vi "Actor Core.vi"(8 "error in":errorcluster, 11 "Jobber in":refnum<class "Jobber.lvclass">) -> (0 "error out":errorcluster, 3 "Actor out":refnum<class "Actor.lvclass">)   [LabVIEW 2014, in "Jobber.lvlib" / "Jobber.lvclass"]
doc: "(<B>Filename</B>: Actor Framework.lvlib:Actor.lvclass:Actor Core.vi)\n\nReceives messages to the actor, reacts to them, and initiates any error handling that may shut the actor down.\n\nDescendant classes may override this VI to append parallel tasks for the actor to complete while it handles messages. Overrides use the Call Parent Method node."
uses:
  Jobber.lvclass
  <vilib>/ActorFramework/Actor/Actor.lvclass
  <vilib>/ActorFramework/Actor/Actor.lvclass/Actor.ctl
  <vilib>/ActorFramework/Message Enqueuer/Message Enqueuer.lvclass/Message Enqueuer.ctl
  Jobber.lvclass/Jobber.ctl
  Shared/Classes/Status Updater/Status Updater.lvclass/Status Updater.ctl
  Jobber Messages/Job Done Msg/Job Done Msg.lvclass/Job Done Msg.ctl
  <vilib>/ActorFramework/Message Enqueuer/Init from Existing Queue.vi
  <vilib>/ActorFramework/Message Enqueuer/Enqueue.vi
  <vilib>/ActorFramework/Message Priority Queue/Priority Enqueue.vi
  Classes/Job/Job.lvclass
  <vilib>/ActorFramework/Message Enqueuer/Message Enqueuer.lvclass
  Jobber Messages/Job Done Msg/Job Done Msg.lvclass
  Shared/Classes/Status Updater/Status Updater.lvclass
panel:
  out "Build Text":string
  out "Progress":u32(slide) scale=0.0..100.0
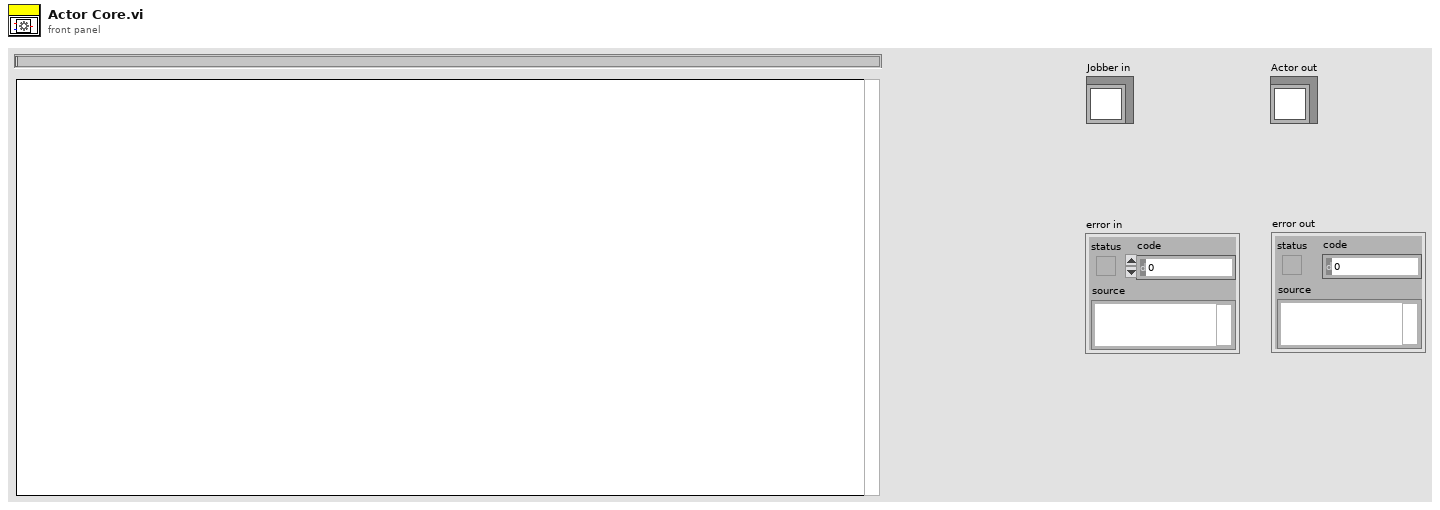
[diagram p1: front panel]
types:
  T1 = enum32{"Invalid", "Standard", "Closed", "Hidden", "Minimized", "Maximized"}
  T2 = cluster{"Event Registration Refnum":refnum<event-registration>, "Event Registration Refnum":refnum<event-registration>}
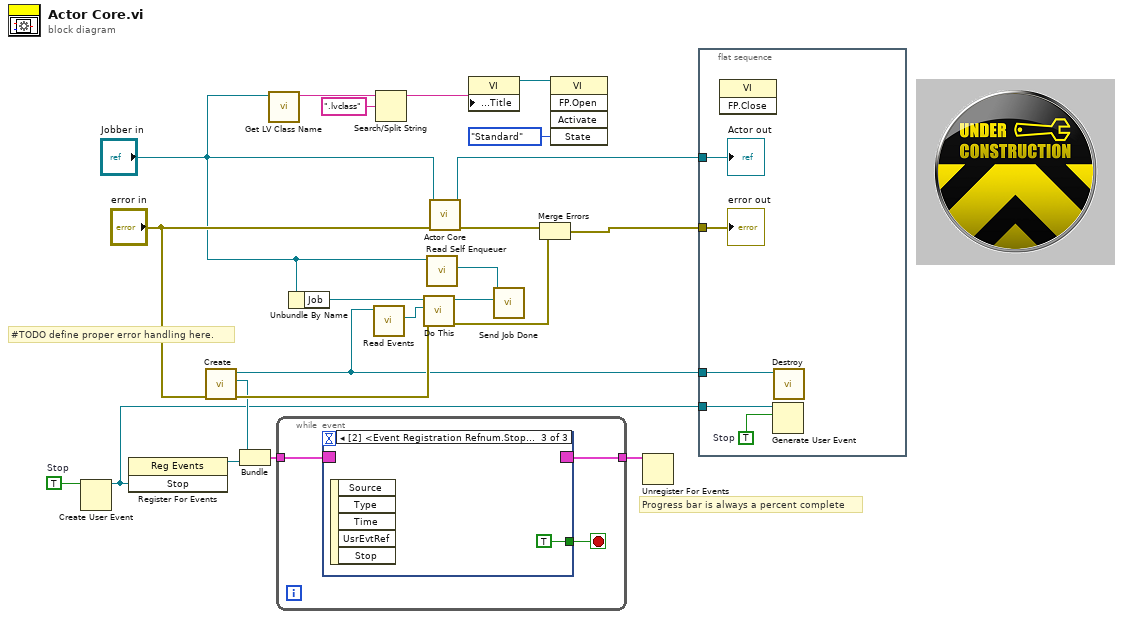
[diagram p0: block diagram]
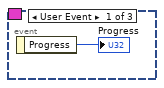
[diagram p2: hidden frame]
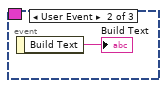
[diagram p3: hidden frame]
diagram:
  w13 = TRUE  # Stop
  # "Progress bar is always a percent complete"
  # "#TODO define proper error handling here."
  n1 = Create User Event(user event datatype=w13) -> (user event=w8:refnum<user-event>)  [unwired: 1 in, 1 out]
  n2 = register-events(w8) -> (reference out=w10:refnum<event-registration>)  [unwired: 2 in, 1 out]
  n3 = call "Create.vi"("error in (no error)"="error in") -> ("error out"=w14:errorcluster, "Event Registration Refnum"=w11:refnum<event-registration>, "Status Updater out"=w9:refnum<class "Status Updater.lvclass">)  [unwired: 8 in]
  n4 = Bundle("Event Registration Refnum"=w11, "Event Registration Refnum"=w10) -> (w12:T2)  [unwired: 1 in]
  n5 = call <vilib>:"Get LV Class Name.vi"("object"="Jobber in") -> ("class name"=w5:string)  [unwired: 9 in, 1 out]
  n6 = while {
    tunnel: w12 -> [w26]
    tunnel: [w24] -> w7
    stop <- w25 stop-if-true
    n7 = event shown="[2] <Event Registration Refnum.Stop>: User Event" {
      selector: w26 -> [_ _ _]
      dyn-events: [_ _ _] -> w24
      timeout: _ -> [_ _ _]
      tunnel: [_ _ TRUE ("Front Panel Window:Closeable")] -> w25
      event User Event {
        n8 = event-data() -> ("Progress"=→"Progress":u32)  [unwired: 1 in]
      }
      event User Event {
        n9 = event-data() -> ("Build Text"=→"Build Text":string)  [unwired: 1 in]
      }
      event User Event {
        n10 = event-data() -> ()  [unwired: 1 in, 5 out]
      }
    }
  }
  n11 = Unbundle By Name("Jobber in") -> ("Job"=w22:refnum<class "Job.lvclass">)
  n12 = call "Read Events.vi"("Status Updater in"=w9) -> ("Status Events"=w16:refnum<class "Status Events.lvclass">)  [unwired: 10 in]
  n13 = Search/Split String(string=w5, search string/char (-)=".lvclass") -> (substring before match=w2:string)  [unwired: 1 in, 2 out]
  n14 = call-dynamic "Do This.vi"("error in (no error)"=w14, "Status Events"=w16, "Job in"=w22) -> ("error out"=w6:errorcluster, "Job out"=w21:refnum<class "Job.lvclass">)  [unwired: 7 in]
  n15 = call <vilib>:"Read Self Enqueuer.vi"("Actor"="Jobber in") -> ("Self Enqueuer"=w20:refnum<class "Message Enqueuer.lvclass">)  [unwired: 10 in]
  n16 = call-parent "Actor Core.vi"("error in"="error in", "Actor in"="Jobber in") -> ("error out"=w19:errorcluster, "Actor out"=w23:refnum<class "Actor.lvclass">)  [unwired: 8 in]
  n17 = property class="VI"("Front Panel.Title"=w2) -> (reference out=w1:refnum<vi>)  [unwired: 2 in, 1 out]
  n18 = call "Send Job Done.vi"("Job"=w21, "Message Enqueuer"=w20) -> ()  [unwired: 8 in, 2 out]
  n19 = Merge Errors(w19, w6) -> (w17:errorcluster)
  n20 = invoke class="VI" method="FP.Open"(reference=w1, "State"=T1."Standard") -> ()  [unwired: 3 in, 5 out]
  n21 = Unregister For Events(event registration refnum=w7) -> ()  [unwired: 1 in, 1 out]
  n22 = flat-sequence {
    tunnel: w23 -> [w34]
    tunnel: w17 -> [w33]
    tunnel: w9 -> [w32]
    tunnel: w8 -> [w30]
    frame #0 {
      w31 = TRUE  # Stop
      n23 = invoke class="VI" method="FP.Close"() -> ()  [unwired: 3 in, 3 out]
      n24 = Generate User Event(user event=w30, event data cluster=w31) -> ()  [unwired: 2 in, 2 out]
      n25 = call "Destroy.vi"("Status Updater in"=w32) -> ()  [unwired: 10 in, 1 out]
      "error out" <- w33
      "Actor out" <- w34
    }
  }
